vi "Launch Actor.vi"(9 "Config Actor":T1, 10 "Actor":refnum<class "Actor.lvclass">) -> (0 "Error out":errorcluster)   [LabVIEW 2025, in "jettl.lvlib" / "Actor.lvlib"]
uses:
  Actor.lvlib
  Actor/Actor.lvclass
  Config Actor.ctl
  Attributes/Attributes/Attributes.lvclass
  Actor.vi
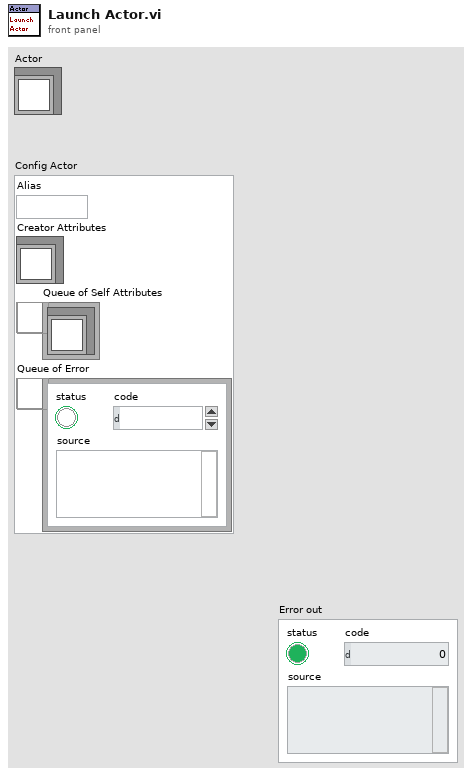
[diagram p1: front panel]
types:
  T1 = typedef "jettl.lvlib/Actor.lvlib/Config Actor.ctl" = cluster{"Alias":string, "Creator Attributes":refnum<class "Attributes.lvclass">, "Queue of Self Attributes":refnum<queue>, "Queue of Error":refnum<queue>}
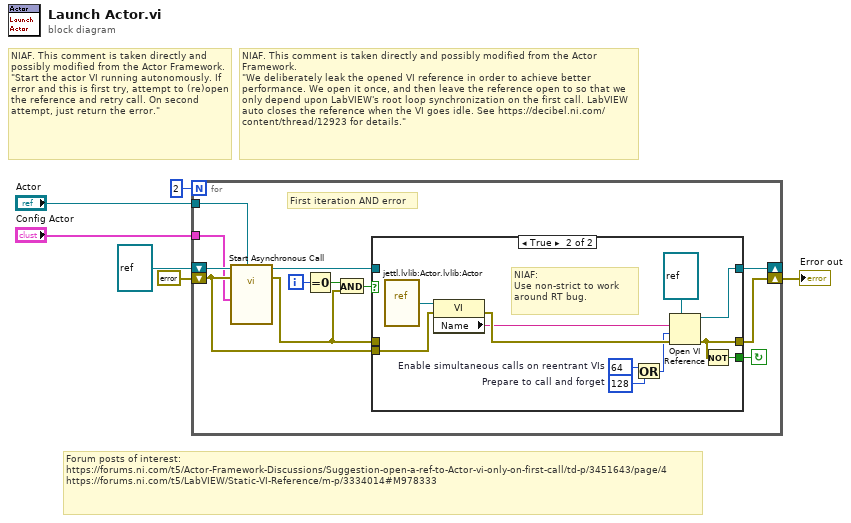
[diagram p0: block diagram]
diagram:
  # "Forum posts of interest:\nhttps://forums.ni.com/t5/Actor-Framework-Discussions/Suggestion-open-a-ref-to-Actor-vi-only-on-first-call/td-p/3451643/page/4\nhttps://forums.ni.com/t5/LabVIEW/Static-VI-Reference/m-p/3334014#M978333"
  # "NIAF. This comment is taken directly and possibly modified from the Actor Framework.\n\"We deliberately leak the opened VI reference in order to achieve better performance. We open it once, and then leave the reference open to so that we only depend upon LabVIEW's root loop synchronization on the first call. LabVIEW auto closes the reference when the VI goes idle. See https://decibel.ni.com/content/thread/12923 for details.\""
  # "NIAF. This comment is taken directly and possibly modified from the Actor Framework.\n\"Start the actor VI running autonomously. If error and this is first try, attempt to (re)open the reference and retry call. On second attempt, just return the error.\""
  n1 = for {
    N: 2 -> [_]
    shift-right: [w18] -> _
    shift-left: refnum<vi> refnum -> [w17]
    shift-right: [w15] -> w3
    shift-left: errorcluster {"status"=FALSE, "code"=0, "source"=""} ("error out") -> [w11]
    tunnel: "Actor" -> [w8]
    tunnel: "Config Actor" -> [w7]
    i -> [w13]
    stop <- w12 continue-if-true
    # "First iteration AND error"
    n2 = call-by-ref "Start Asynchronous Call"(reference=w17, error in=w11, "Actor in"=w8, "Config Actor"=w7) -> (reference out=w16:refnum<vi>, error out=w9:errorcluster)  [unwired: 8 in, 2 out]
    n3 = Equal To 0?(x=w13) -> (x = 0?=w10:bool)
    n4 = And(x=w10, y=w9) -> (x .and. y?=w14:bool)
    n5 = case shown="True" w14 {
      tunnel: [w20 w29] -> w18
      tunnel: [w19 w27] -> w15
      tunnel: w16 -> [w20 _]
      tunnel: w9 -> [w19 _]
      tunnel: [_ w28] -> w12
      tunnel: w11 -> [_ w26]
      frame False {
      }
      frame True {
        w21 = 64  # Enable simultaneous calls on reentrant VIs
        w23 = 128  # Prepare to call and forget
        # "NIAF:\nUse non-strict to work around RT bug."
        n6 = vi-ref "jettl.lvlib:Actor.lvlib:Actor.vi"() -> (w25:refnum<vi>)
        n7 = property class="VI"(reference=w25, error in=w26) -> (error out=w31:errorcluster, "Name"=w30:string)  [unwired: 1 out]
        n8 = Or(x=w21, y=w23) -> (x .or. y?=w22:i32)
        n9 = Open VI Reference(type specifier VI Refnum (for type only)=refnum<vi> refnum, vi path=w30, options=w22, error in (no error)=w31) -> (vi reference=w29:refnum<vi>, error out=w27:errorcluster)  [unwired: 2 in]
        n10 = Not(x=w27) -> (.not. x?=w28:bool)
      }
    }
  }
  "Error out" <- w3
